vi "Simulator VNA Unflatten Driver Configuration.vi"(9 "VNA Configuration (\"\")":string) -> (1 "Configuration":T1={"BusType"=enum."GPIB", "GPIB Bus"=0, "GPIB Address"=0, "IP"=0, "COM"=0, "Baud Rate"=enum."300", "USB Device"=0, "Instrument S\\N"="", "SCIL Address"=16} {"USB Device" max=31 step=1}, 4 "Version":string)   [LabVIEW 2011]
uses:
  VNA Configuration.ctl
  VNA Configuration v1.ctl
  VNA Configuration v2.ctl
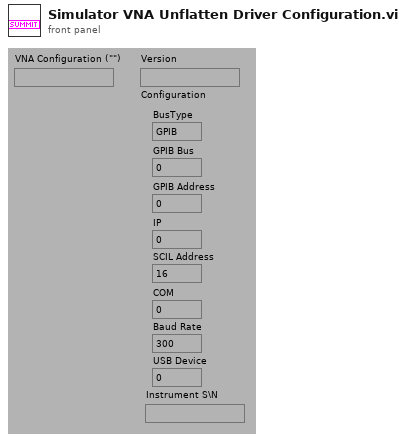
[diagram p1: front panel]
types:
  T1 = typedef "VNA Configuration.ctl" = cluster{"BusType":enum32{"GPIB", "LAN/IP", "Serial", "USB"}, "GPIB Bus":i32, "GPIB Address":i32, "IP":u32, "COM":i32, "Baud Rate":enum32{"300", "600", "1200", "2400", "4800", "9600"}, "USB Device":u32, "Instrument S\\N":string, "SCIL Address":i32}
  T2 = typedef "VNA Configuration v1.ctl" = cluster{"BusType":enum32{"GPIB", "LAN/IP", "Serial", "USB"}, "GPIB Bus":i32, "GPIB Address":i32, "IP":u32, "COM":i32, "Baud Rate":enum32{"300", "600", "1200", "2400", "4800", "9600"}}
  T3 = typedef "VNA Configuration v2.ctl" = cluster{"BusType":enum32{"GPIB", "LAN/IP", "Serial", "USB"}, "GPIB Bus":i32, "GPIB Address":i32, "IP":u32, "COM":i32, "Baud Rate":enum32{"300", "600", "1200", "2400", "4800", "9600"}, "USB Device":u32, "Instrument S\\N":string}
  T4 = enum32{"300", "600", "1200", "2400", "4800", "9600"}
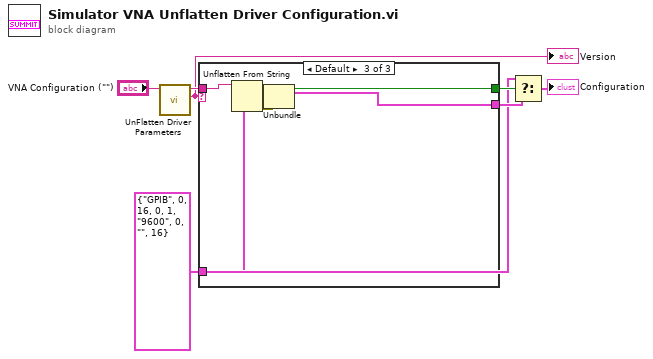
[diagram p0: block diagram]
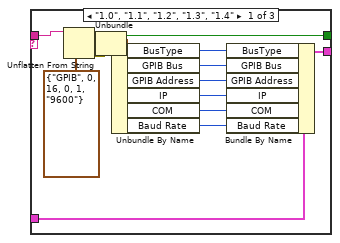
[diagram p2: hidden frame]
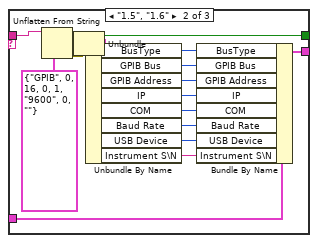
[diagram p3: hidden frame]
diagram:
  w2 = T1 {"BusType"=enum."GPIB", "GPIB Bus"=0, "GPIB Address"=16, "IP"=0, "COM"=1, "Baud Rate"=enum."9600", "USB Device"=0, "Instrument S\\N"="", "SCIL Address"=16} ("Configuration")
  n1 = call "UnFlatten Driver Parameters.vi"("Flattened Driver Parameters with Version (\"\")"="VNA Configuration (\"\")") -> ("Driver Version"=w1:string, "Flat Driver Parameters"=w3:string)  [unwired: 1 in, 4 out]
  "Version" <- w1
  n2 = case shown="Default" w1 {
    tunnel: [w16 w31 w40] -> w7
    tunnel: [w20 w35 w39] -> w5
    tunnel: w3 -> [w19 w34 w38]
    tunnel: w2 -> [w17 w32 w37]
    frame "1.0", "1.1", "1.2", "1.3", "1.4" {
      n3 = Unflatten From String(type=T2 {"BusType"=enum."GPIB", "GPIB Bus"=0, "GPIB Address"=16, "IP"=0, "COM"=1, "Baud Rate"=enum."9600"} ("Configuration"), binary string=w19) -> (value=w15:T2, error out=w8:errorcluster)  [unwired: 1 in, 3 out]
      n4 = Unbundle(w8) -> ("status"=w20:bool)  [unwired: 2 out]
      n5 = Unbundle By Name(w15) -> ("BusType"=w14:enum32{"GPIB", "LAN/IP", "Serial", "USB"}, "GPIB Bus"=w13:i32, "GPIB Address"=w12:i32, "IP"=w11:u32, "COM"=w10:i32, "Baud Rate"=w9:T4)
      n6 = Bundle By Name(cluster=w17, "BusType"=w14, "GPIB Bus"=w13, "GPIB Address"=w12, "IP"=w11, "COM"=w10, "Baud Rate"=w9) -> (w16:T1)
    }
    frame "1.5", "1.6" {
      n7 = Unflatten From String(type=T3 {"BusType"=enum."GPIB", "GPIB Bus"=0, "GPIB Address"=16, "IP"=0, "COM"=1, "Baud Rate"=enum."9600", "USB Device"=0, "Instrument S\\N"=""} ("Configuration"), binary string=w34) -> (value=w30:T3, error out=w21:errorcluster)  [unwired: 1 in, 3 out]
      n8 = Unbundle(w21) -> ("status"=w35:bool)  [unwired: 2 out]
      n9 = Unbundle By Name(w30) -> ("BusType"=w29:enum32{"GPIB", "LAN/IP", "Serial", "USB"}, "GPIB Bus"=w28:i32, "GPIB Address"=w27:i32, "IP"=w26:u32, "COM"=w25:i32, "Baud Rate"=w24:T4, "USB Device"=w23:u32, "Instrument S\\N"=w22:string)
      n10 = Bundle By Name(cluster=w32, "BusType"=w29, "GPIB Bus"=w28, "GPIB Address"=w27, "IP"=w26, "COM"=w25, "Baud Rate"=w24, "USB Device"=w23, "Instrument S\\N"=w22) -> (w31:T1)
    }
    frame Default {
      n11 = Unflatten From String(type=w37, binary string=w38) -> (value=w40:T1, error out=w36:errorcluster)  [unwired: 1 in, 3 out]
      n12 = Unbundle(w36) -> ("status"=w39:bool)  [unwired: 2 out]
    }
  }
  n13 = Select(t=w2, s=w5, f=w7) -> (s? t:f=→"Configuration":T1)
